vi "runtest Save Test Run.vi"(7 "Test Output":T4, 8 "error in (no error)":errorcluster, 9 "Wait for Organization? (f)":bool, 10 "Overwrite Existing? (f)":bool, 11 "Fields In":T1[](array[typedef])) -> (0 "error out":errorcluster, 1 "Run ID String":string, 2 "Data File Path":path, 3 "Fields Out":T1[](array[typedef]))   [LabVIEW 2011]
uses:
  server/database/Fields/Field Record.ctl
  server/database/Fields/Field DataTypes.ctl
  server/database/Fields/Field NextItem.ctl
  tests/Test Output.ctl
  server/database/Fields/Field System Fields.ctl
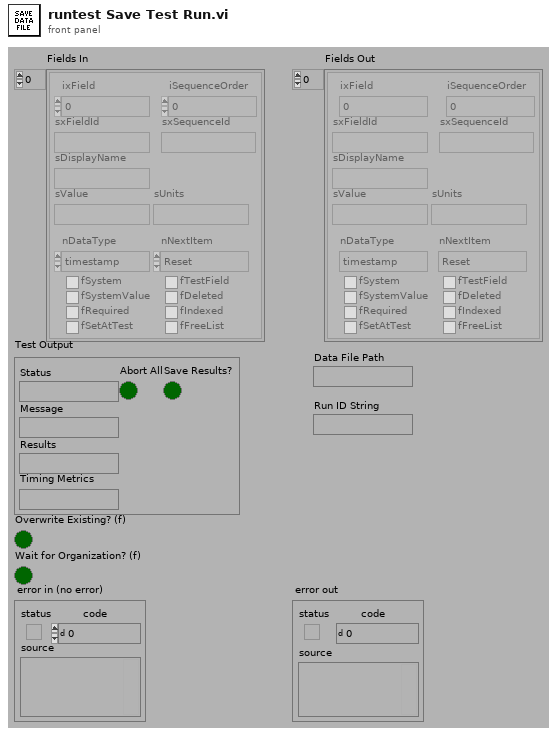
[diagram p1: front panel]
types:
  T1 = typedef "Field Record.ctl" = cluster{"ixField":i32, "iSequenceOrder":i32, "sxFieldId":string, "sxSequenceId":string, "sDisplayName":string, "sValue":string, "sUnits":string, "nDataType":T2, "nNextItem":T3, "fSystem":bool, "fSystemValue":bool, "fRequired":bool, "fSetAtTest":bool, "fTestField":bool, "fDeleted":bool, "fIndexed":bool, "fFreeList":bool}
  T2 = typedef "Field DataTypes.ctl" = enum32{"text", "numeric", "list", "timestamp", "boolean"}
  T3 = typedef "Field NextItem.ctl" = enum32{"Reset", "Retain", "Auto-Increment"}
  T4 = typedef "Test Output.ctl" = cluster{"Status":string, "Message":string, "Results":string, "Abort All":bool, "Save Results?":bool, "Timing Metrics":string}
  T5 = enum16{"open", "open or create", "create or replace", "create", "open (read-only)"}
  T6 = typedef "Field System Fields.ctl" = enum32{"Company", "End_Timestamp", "Model_Number", "Operator", "Serial_Number", "Start_Timestamp", "Step_Number", "Step_Tag", "Test_Run", "Test_Sequence", "Test_Station", "Test_Station_Name", "Test_Status", "Test_Type", "Test_Version", "Spartan_Version_Created", "Spartan_Version_Current"}
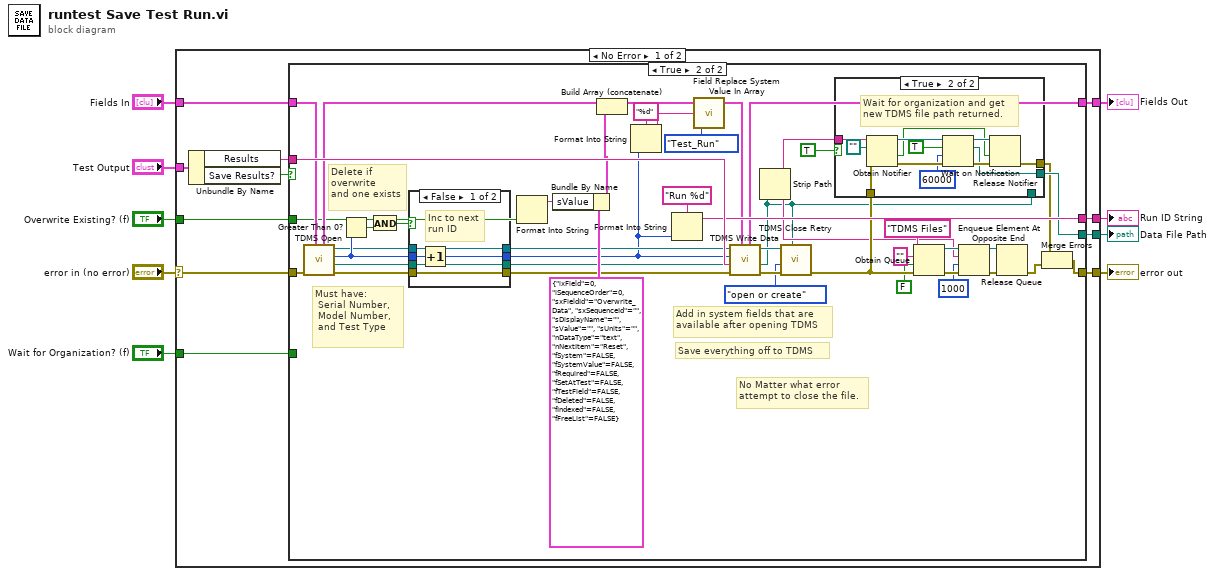
[diagram p0: block diagram]
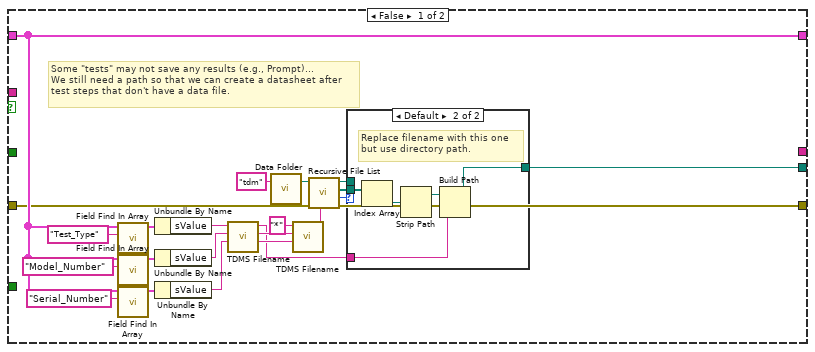
[diagram p2: hidden frame]
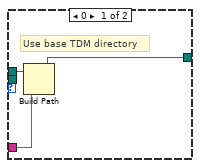
[diagram p3: hidden frame]
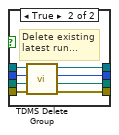
[diagram p5: hidden frame]
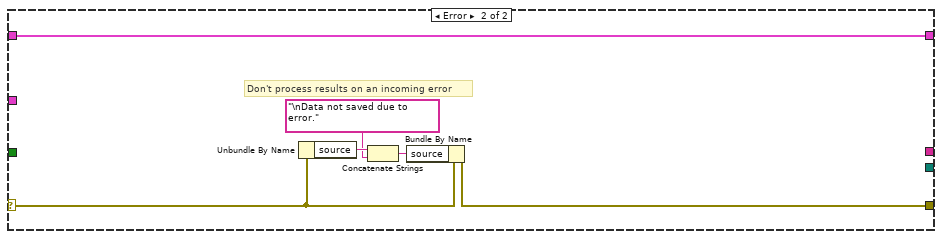
[diagram p6: hidden frame]
diagram:
  n1 = case shown="No Error" "error in (no error)" {
    selector: "error in (no error)" -> [w19 w124]
    tunnel: [w20 w125] -> w9
    tunnel: "Test Output" -> [w17 _]
    tunnel: "Fields In" -> [w16 w126]
    tunnel: [w15 _] -> w5
    tunnel: [w14 _] -> w4
    tunnel: "Overwrite Existing? (f)" -> [w13 _]
    tunnel: [w11 w126] -> w2
    tunnel: "Wait for Organization? (f)" -> [w10 _]
    frame No Error {
      n2 = Unbundle By Name(w17) -> ("Results"=w18:string, "Save Results?"=w12:bool)
      n3 = case shown="True" w12 {
        tunnel: [w31 w53] -> w20
        tunnel: w19 -> [w32 w92]
        tunnel: w16 -> [w35 w91]
        tunnel: w18 -> [_ w93]
        tunnel: w13 -> [_ w83]
        tunnel: [w22 w57] -> w14
        tunnel: [_ w90] -> w15
        tunnel: [w35 w89] -> w11
        tunnel: w10 -> [_ _]
        frame False {
          # "Some \"tests\" may not save any results (e.g., Prompt)...\nWe still need a path so that we can create a datasheet after\ntest steps that don't have a data file."
          n4 = call "Field Find In Array.vi"("FieldID or Display Name(\"\")"="Test_Type" ("Field Internal ID"), "Field Array"=w35) -> ("Field"=w41:T1)  [unwired: 1 in, 8 out]
          n5 = call "Field Find In Array.vi"("FieldID or Display Name(\"\")"="Model_Number" ("Field Internal ID"), "Field Array"=w35) -> ("Field"=w36:T1)  [unwired: 1 in, 8 out]
          n6 = call "Field Find In Array.vi"("FieldID or Display Name(\"\")"="Serial_Number" ("Field Internal ID"), "Field Array"=w35) -> ("Field"=w37:T1)  [unwired: 1 in, 8 out]
          n7 = Unbundle By Name(w41) -> ("sValue"=w34:string)
          n8 = Unbundle By Name(w36) -> ("sValue"=w30:string)
          n9 = Unbundle By Name(w37) -> ("sValue"=w29:string)
          n10 = call "TDMS Filename.vi"("Serial Number"=w29, "Model Number"=w30, "Test Type"=w34) -> ("Filename"=w24:string)  [unwired: 8 out]
          n11 = call "Data Folder.vi"("Relative Path (\"\" - Folder)"="tdm") -> ("Data Folder"=w23:path)  [unwired: 2 in]
          n12 = call "TDMS Filename.vi"("Serial Number"=w29, "Model Number"=w30, "Test Type"="*" ("Field Internal ID")) -> ("Filename"=w27:string)  [unwired: 8 out]
          n13 = call <vilib>:"Recursive File List.vi"("pattern"=w27, "error in (no error)"=w32, "Folder Path"=w23) -> ("error out"=w31:errorcluster, "Number of Files"=w26:i32, "All Files in Dir"=w21:path[], "dup Folder Path"=w25:path)  [unwired: 4 in, 1 out]
          n14 = case shown="Default" w26 {
            tunnel: w25 -> [w44 _]
            tunnel: w24 -> [w43 w49]
            tunnel: [w42 w48] -> w22
            tunnel: w21 -> [_ w47]
            frame 0 {
              # "Use base TDM directory"
              n15 = Build Path(base path=w44, name or relative path=w43) -> (appended path=w42:path)
            }
            frame Default {
              # "Replace filename with this one\nbut use directory path."
              n16 = Index Array(array=w47) -> (element=w45:path)  [unwired: 1 in]
              n17 = Strip Path(path=w45) -> (stripped path=w46:path)  [unwired: 1 out]
              n18 = Build Path(base path=w46, name or relative path=w49) -> (appended path=w48:path)
            }
          }
        }
        frame True {
          # "Add in system fields that are\navailable after opening TDMS"
          # "Save everything off to TDMS"
          # "Must have: \n Serial Number, \n Model Number,\n and Test Type"
          # "No Matter what error\nattempt to close the file."
          # "Delete if\noverwrite\nand one exists"
          n19 = call "TDMS Open.vi"("Fields In"=w91, "error in (no error)"=w92) -> ("error out"=w87:errorcluster, "TDMS File Path"=w86:path, "Last Run #"=w85:i32, "TDMS File Ref"=w84:refnum<k34>, "Fields Out"=w88:T1[])  [unwired: 1 in, 4 out]
          n20 = Greater Than 0?(x=w85) -> (x > 0?=w80:bool)
          n21 = And(x=w83, y=w80) -> (x .and. y?=w62:bool)
          n22 = case shown="False" w62 {
            tunnel: w87 -> [w112 w120]
            tunnel: [w112 w119] -> w63
            tunnel: w85 -> [w110 w114]
            tunnel: [w109 w113] -> w64
            tunnel: [w111 w117] -> w65
            tunnel: w84 -> [w111 w118]
            tunnel: w86 -> [w108 w116]
            tunnel: [w108 w115] -> w58
            frame False {
              # "Inc to next\nrun ID"
              n23 = Increment(x=w110) -> (x+1=w109:i32)
            }
            frame True {
              # "Delete existing\nlatest run..."
              n24 = call "TDMS Delete Group.vi"("error in (no error)"=w120, "File Path In"=w116, "Run to Delete"=w114, "TDMS File Ref"=w118) -> ("error out"=w119:errorcluster, "File Path Out"=w115:path, "Run #"=w113:i32, "TDMS File Ref"=w117:refnum<k34>)  [unwired: 1 in, 3 out]
            }
          }
          n25 = Format Into String(w83) -> (resulting string=w73:string)  [unwired: 3 in, 1 out]
          n26 = Bundle By Name(cluster=T1 {"ixField"=0, "iSequenceOrder"=0, "sxFieldId"="Overwrite_Data", "sxSequenceId"="", "sDisplayName"="", "sValue"="", "sUnits"="", "nDataType"=enum."text", "nNextItem"=enum."Reset", "fSystem"=FALSE, "fSystemValue"=FALSE, "fRequired"=FALSE, "fSetAtTest"=FALSE, "fTestField"=FALSE, "fDeleted"=FALSE, "fIndexed"=FALSE, "fFreeList"=FALSE} ("Field Record"), "sValue"=w73) -> (w70:T1)
          n27 = Build Array (concatenate)(w88, w70) -> (w72:T1[])
          n28 = Format Into String(format string="%d", w64) -> (resulting string=w75:string)  [unwired: 2 in, 1 out]
          n29 = Format Into String(format string="Run %d", w64) -> (resulting string=w90:string)  [unwired: 2 in, 1 out]
          n30 = call "Field Replace System Value In Array.vi"("System Field to Replace (Serial Number)"=Field_System_Fields."Test_Run", "Field Value Replacement Data (\"\")"=w75, "Fields Array In"=w72) -> ("Fields Array Out"=w74:T1[])  [unwired: 1 in, 1 out]
          n31 = call "TDMS Write Data.vi"("Fields Array In"=w74, "error in (no error)"=w63, "Test Results (\"\")"=w93, "Test Run (1)"=w64, "TDMS File Ref"=w65) -> ("error out"=w78:errorcluster, "TDMS File Ref"=w79:refnum<k34>, "Fields Array Out"=w89:T1[])  [unwired: 1 in, 3 out]
          n32 = Strip Path(path=w58) -> (name=w59:string)  [unwired: 1 out]
          n33 = call "TDMS Close Retry.vi"("TDMS Path"=w58, "error in (no error)"=w78, "Operation (0:open)"=T5."open or create" ("operation (0:open)"), "TDMS File Ref"=w79) -> ("error out"=w60:errorcluster)  [unwired: 1 in, 6 out]
          n34 = case shown="True" TRUE {
            tunnel: w60 -> [w94 w105]
            tunnel: w59 -> [_ w101]
            tunnel: [w95 w98] -> w57
            tunnel: w58 -> [w95 _]
            tunnel: [w94 w96] -> w55
            frame False {
              # "Don't wait for organization."
            }
            frame True {
              # "Wait for organization and get\nnew TDMS file path returned."
              n35 = Obtain Notifier(name (unnamed)=w101, notification data type=path "", error in (no error)=w105) -> (notifier out=w104:refnum<notifier>, created new?=w100:bool, error out=w107:errorcluster)  [unwired: 1 in]
              n36 = Wait on Notification(notifier=w104, ignore previous (F)=TRUE, timeout in ms (-1)=60000, error in (no error)=w107) -> (notifier out=w103:refnum<notifier>, notification=w98:path, error out=w106:errorcluster)  [unwired: 1 out]
              n37 = Release Notifier(notifier=w103, force destroy? (F)=w100, error in (no error)=w106) -> (error out=w96:errorcluster)  [unwired: 2 out]
            }
          }
          n38 = Obtain Queue(name (unnamed)="TDMS Files", element data type="", create if not found? (T)=FALSE, error in (no error)=w60) -> (queue out=w66:refnum<queue>, error out=w67:errorcluster)  [unwired: 1 in, 1 out]
          n39 = Enqueue Element At Opposite End(queue=w66, element=w59, timeout in ms (-1)=1000, error in (no error)=w67) -> (queue out=w51:refnum<queue>, error out=w52:errorcluster)  [unwired: 1 out]
          n40 = Release Queue(queue=w51, error in (no error)=w52) -> (error out=w54:errorcluster)  [unwired: 1 in, 2 out]
          n41 = Merge Errors(w55, w54) -> (w53:errorcluster)
        }
      }
    }
    frame Error {
      # "Don't process results on an incoming error"
      n42 = Unbundle By Name(w124) -> ("source"=w123:string)
      n43 = Concatenate Strings(w123, "\nData not saved due to error." ("name (unnamed)")) -> (w121:string)
      n44 = Bundle By Name(cluster=w124, "source"=w121) -> (w125:errorcluster)
    }
  }
  "error out" <- w9
  "Data File Path" <- w4
  "Run ID String" <- w5
  "Fields Out" <- w2
